vi "read_mic.vi"() -> ()   [LabVIEW 2014]
uses:
  <vilib>/sound2/lvsound2.llb/Sampling Mode.ctl
  <vilib>/sound2/lvsound2.llb/Sound Data Format.ctl
  <vilib>/sound2/lvsound2.llb/Sound Input Read (DBL).vi
  <vilib>/sound2/lvsound2.llb/Sound Output Write (DBL Single).vi
panel:
  in  "stop 2":bool
  out "Waveform Graph":waveform(dbl)(graph)
  in  "stop":bool
  in  "Input Device ID":u32
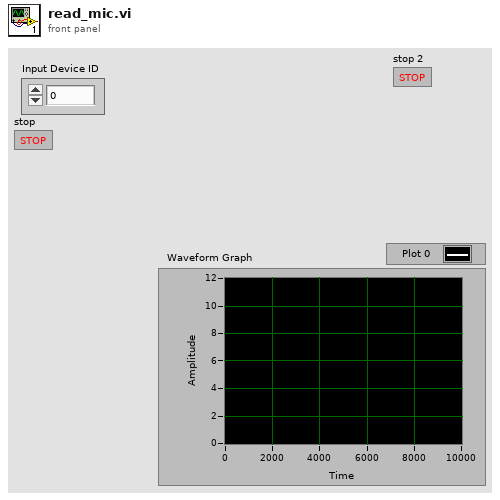
[diagram p1: front panel]
types:
  T1 = typedef "Sound Data Format.ctl" = cluster{"sample rate (S/s)":dbl, "number of channels":i32, "bits per sample":i32}
  T2 = typedef "Sampling Mode.ctl" = i32
  T3 = typedef "Sound Input Task ID.ctl" = u32
  T4 = typedef "Sound Output Task ID.ctl" = u32
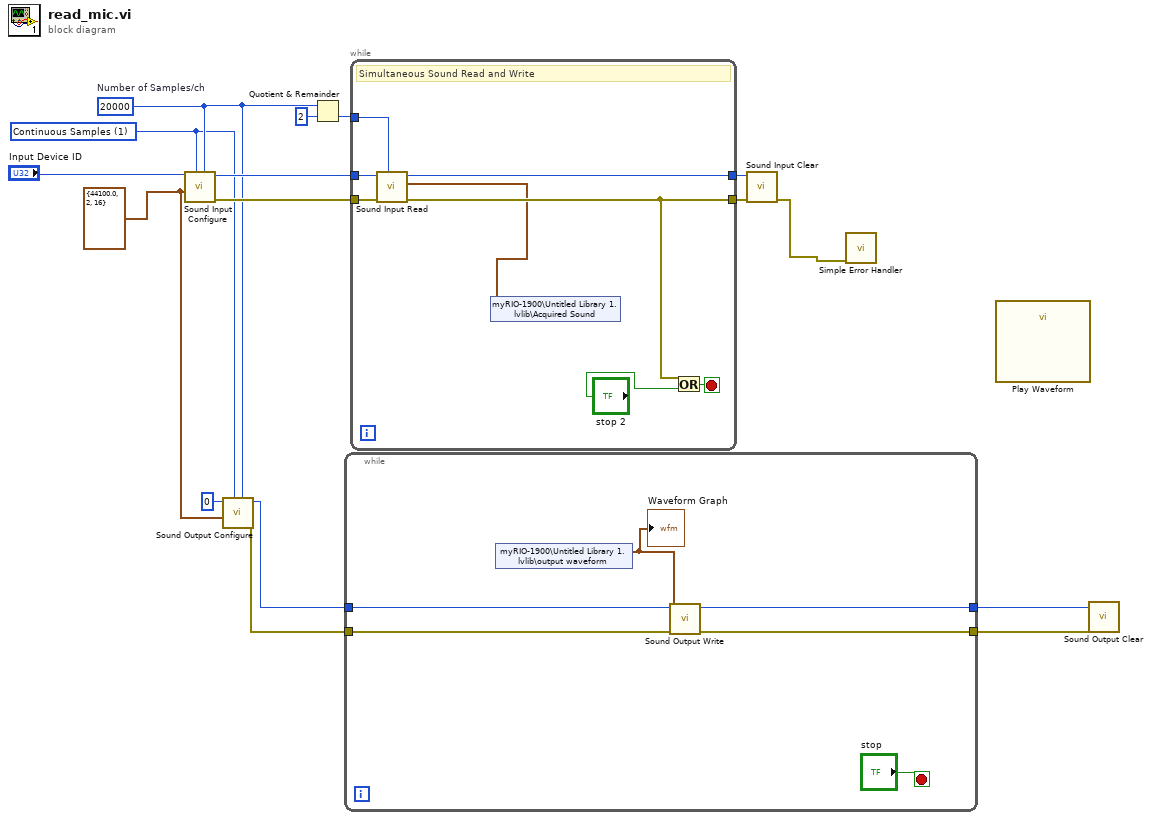
[diagram p0: block diagram]
diagram:
  w7 = 20000  # Number of Samples/ch
  w8 = T1 {"sample rate (S/s)"=44100.0, "number of channels"=2, "bits per sample"=16} ("Sound Format")
  w6 = T2 1 items=["Finite Samples", "Continuous Samples"] ("sample mode")
  n1 = call <vilib>:"Sound Input Configure.vi"("number of samples/ch"=w7, "sample mode"=w6, "sound format"=w8, "device ID"="Input Device ID") -> ("error out"=w13:errorcluster, "task ID"=w12:T3)  [unwired: 6 in]
  n2 = call <vilib>:"Sound Output Configure.vi"("number of samples/ch"=w7, "sample mode"=w6, "sound format"=w8, "device ID"=u32 0) -> ("error out"=w1:errorcluster, "task ID"=w4:T4)  [unwired: 6 in]
  n3 = Quotient & Remainder(x=w7, y=2) -> (floor(x/y)=w11:i32)  [unwired: 1 out]
  n4 = while {
    tunnel: w4 -> [w21]
    tunnel: [w19] -> w3
    tunnel: [w18] -> w2
    tunnel: w1 -> [w17]
    stop <- "stop" stop-if-true
    n5 = shared-variable "myRIO-1900\\Untitled Library 1.lvlib\\output waveform"() -> (w20:waveform(dbl))  [unwired: 1 in, 1 out]
    "Waveform Graph" <- w20
    n6 = call-poly <vilib>:"Sound Output Write.vi"("error in (no error)"=w17, "data"=w20, "task ID"=w21) -> ("error out"=w19:errorcluster, "task ID out"=w18:T4)  [unwired: 7 in]
  }
  n7 = while {
    tunnel: w11 -> [w28]
    tunnel: w12 -> [w29]
    tunnel: [w27] -> w14
    tunnel: w13 -> [w30]
    tunnel: [w26] -> w16
    stop <- w25 stop-if-true
    # "Simultaneous Sound Read and Write"
    n8 = call-poly <vilib>:"Sound Input Read.vi"("number of samples/ch"=w28, "error in (no error)"=w30, "task ID"=w29) -> ("error out"=w26:errorcluster, "data"=w24:waveform(dbl)[], "task ID out"=w27:T3)  [unwired: 6 in]
    n9 = shared-variable "myRIO-1900\\Untitled Library 1.lvlib\\Acquired Sound"(w24) -> ()  [unwired: 1 in, 1 out]
    n10 = Or(x=w26, y="stop 2") -> (x .or. y?=w25:bool)
  }
  n11 = call <vilib>:"Sound Input Clear.vi"("error in (no error)"=w16, "task ID"=w14) -> ("error out"=w9:errorcluster)  [unwired: 9 in]
  n12 = call <vilib>:"Simple Error Handler.vi"("error in (no error)"=w9) -> ()  [unwired: 4 in, 5 out]
  n13 = call "Play Waveform"() -> ()  [unwired: 19 in, 1 out]
  n14 = call <vilib>:"Sound Output Clear.vi"("error in (no error)"=w3, "task ID"=w2) -> ()  [unwired: 9 in, 1 out]
